vi "Initialize DAQ parameters.vi"(8 "error in":errorcluster, 10 "DAQ Input Parameters":T1={"Mode"=enum."Scanning", "Zoom"=0, "Acceptance Angle"=0, "AOD fill"=0, "Wavelength"=0, "Speed of Sound(Va)"=0, "Samps-per-pix(P)"=0, "Numer-pixels-pointing(Np)"=0, "Samples Wait after Trigger"=0, "StartUp Delay"=0, "x-pixels-per-line(NPx) (fast)"=0, "y-pixels-per-line(NPy) (slow)"=0, "Repeat (Number of Cycles)"=0, "Number of Trials"=0, "Slip Cycle"=163840, "Use accumulate green"=FALSE, "Use accumulate red"=FALSE, "Add Cycle"=FALSE, "accn_noise"=6000.0, "var_y"=1.0, "var_x"=1.0, "New line trigger enabled"=FALSE} {"var_x" format="%#_14g"; "var_y" format="%#_14g"}, 11 "FPGA VI Reference":T3) -> (0 "error out":errorcluster, 3 "FPGA VI Reference":T3)   [LabVIEW 2017]
uses:
  RIG-SPECIFIC FILES/FPGA Refs/FPGA Ref.ctl
  Typedefs/Controls/DAQ Input Parameters(FlexRIO).ctl
  FPGA Typedefs/scan_typr.ctl
  <vilib>/Utility/error.llb/Error Cluster From Error Code.vi
  <vilib>/rvi/errors/niLvFpgaAdjustHostInterfaceError.vi
  <vilib>/rvi/interface/nirviReadWriteControl/nirviReadWriteControl.xnode
  NiFpgaLv.dll
  <vilib>/rvi/interface/Simulation/niFpgaSimulationCallBeginRW.vi
panel:
  in  "bg_cycles":u16=40
  out "samples wait after pulse":u16=6050
  out "Samples Wait after Trigger":u16=5843
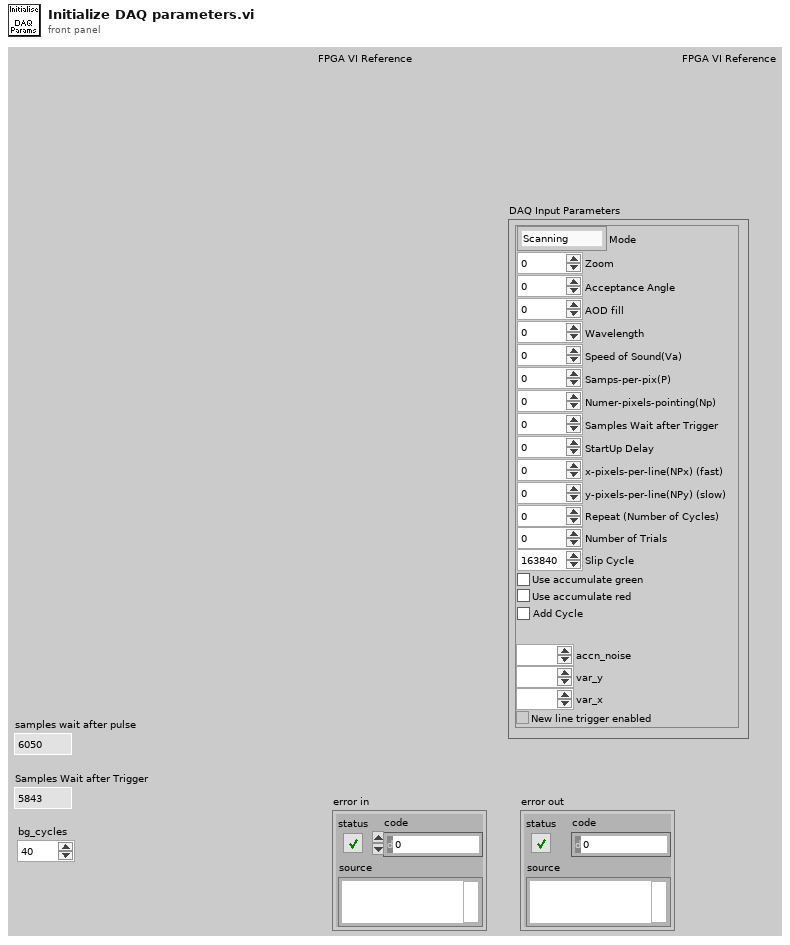
[diagram p1: front panel]
types:
  T1 = typedef "DAQ Input Parameters(FlexRIO).ctl" = cluster{"Mode":T2, "Zoom":i8, "Acceptance Angle":i8, "AOD fill":u16, "Wavelength":i16, "Speed of Sound(Va)":i8, "Samps-per-pix(P)":i16, "Numer-pixels-pointing(Np)":u32, "Samples Wait after Trigger":u16, "StartUp Delay":i32, "x-pixels-per-line(NPx) (fast)":u16, "y-pixels-per-line(NPy) (slow)":u16, "Repeat (Number of Cycles)":u32, "Number of Trials":u16, "Slip Cycle":u32, "Use accumulate green":bool, "Use accumulate red":bool, "Add Cycle":bool, "accn_noise":fxp<+,16,16>, "var_y":fxp<+,16,4>, "var_x":fxp<+,16,4>, "New line trigger enabled":bool}
  T2 = typedef "scan_typr.ctl" = enum16{"Scanning", "Pointing", "Pointing & MC", "Scanning & MC"}
  T3 = typedef "FPGA Ref.ctl" = refnum<k20>
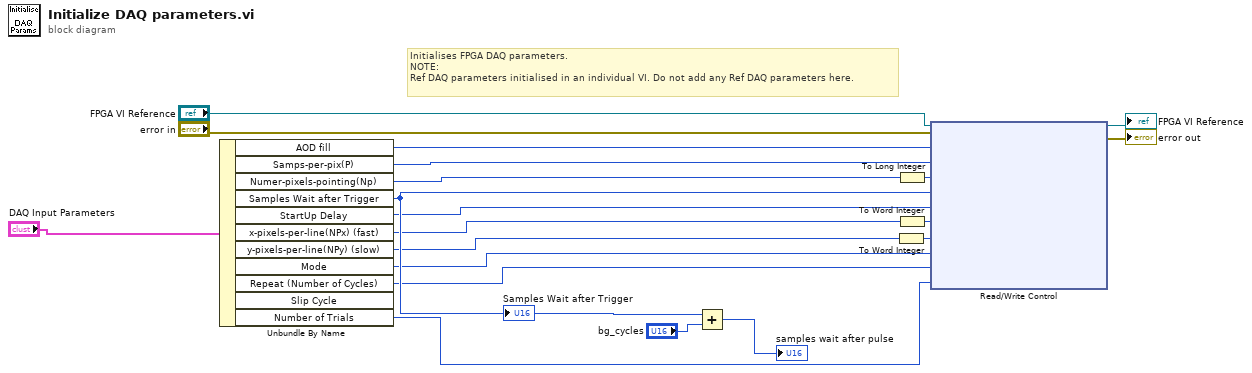
[diagram p0: block diagram]
diagram:
  # "Initialises FPGA DAQ parameters.\nNOTE:\nRef DAQ parameters initialised in an individual VI. Do not add any Ref DAQ parameters here."
  n1 = Unbundle By Name("DAQ Input Parameters") -> ("AOD fill"=w15:u16, "Samps-per-pix(P)"=w14:i16, "Numer-pixels-pointing(Np)"=w8:u32, "Samples Wait after Trigger"=w18:u16, "StartUp Delay"=w13:i32, "x-pixels-per-line(NPx) (fast)"=w12:u16, "y-pixels-per-line(NPy) (slow)"=w11:u16, "Mode"=w5:T2, "Repeat (Number of Cycles)"=w10:u32, "Number of Trials"=w2:u16)  [unwired: 1 out]
  "Samples Wait after Trigger" <- w18
  n2 = Add(x=w18, y="bg_cycles") -> (x+y=→"samples wait after pulse":u16)
  n3 = To Word Integer(number=w11) -> (16bit integer=w16:i16)
  n4 = To Long Integer(number=w8) -> (32bit integer=w9:i32)
  n5 = To Word Integer(number=w12) -> (16bit integer=w17:i16)
  n6 = xnode "Read/Write Control"("FPGA VI Reference In"="FPGA VI Reference", "error in"="error in", "AOD fill"=w15, "samps-per-pix (P)"=w14, "Number-pixels-pointing (Np)"=w9, "samples wait after trigger"=w18, "Start Up Delay"=w13, "x-pixels-per-line (Npx)"=w17, "y-pixels-per-line (Npy)"=w16, "Mode"=w5, "Repeat (Number of Cycles)"=w10, "trial_num_trial"=w2) -> ("FPGA VI Reference Out"=→"FPGA VI Reference":T3, "error out"=→"error out":errorcluster)
